vi "pwm_analog_digital.vi"() -> ()   [LabVIEW 2018]
uses:
  <vilib>/Instr/_visa.llb/VISA Configure Serial Port (Instr).vi
panel:
  in  "Boolean":bool
  out "concatenated string":string
  in  "Slide":dbl(slide) scale=0.0..255.0
  out "x = y?":bool
  in  "stop":bool
  out "Gauge":dbl(knob)
  in  "VISA resource name":refnum<visa-resource-name>
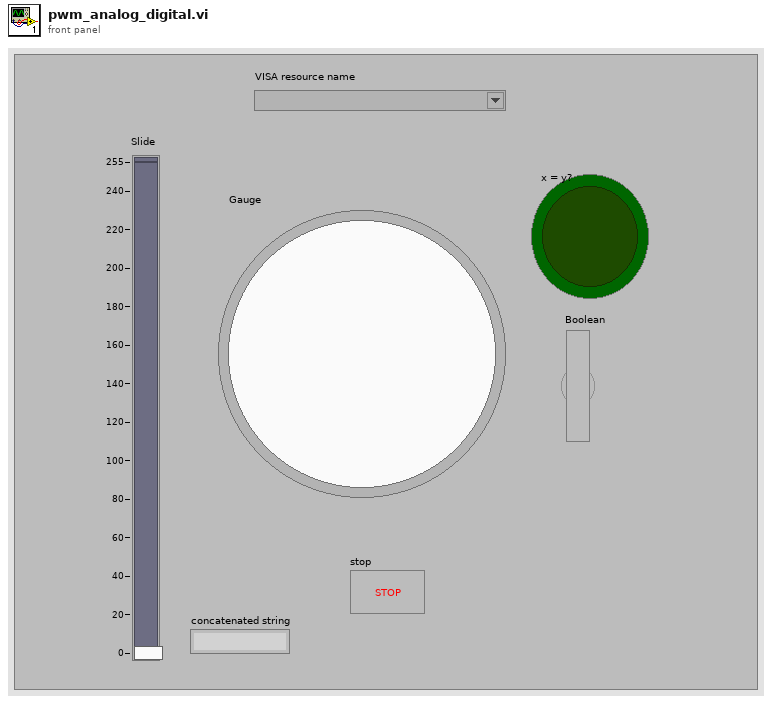
[diagram p1: front panel]
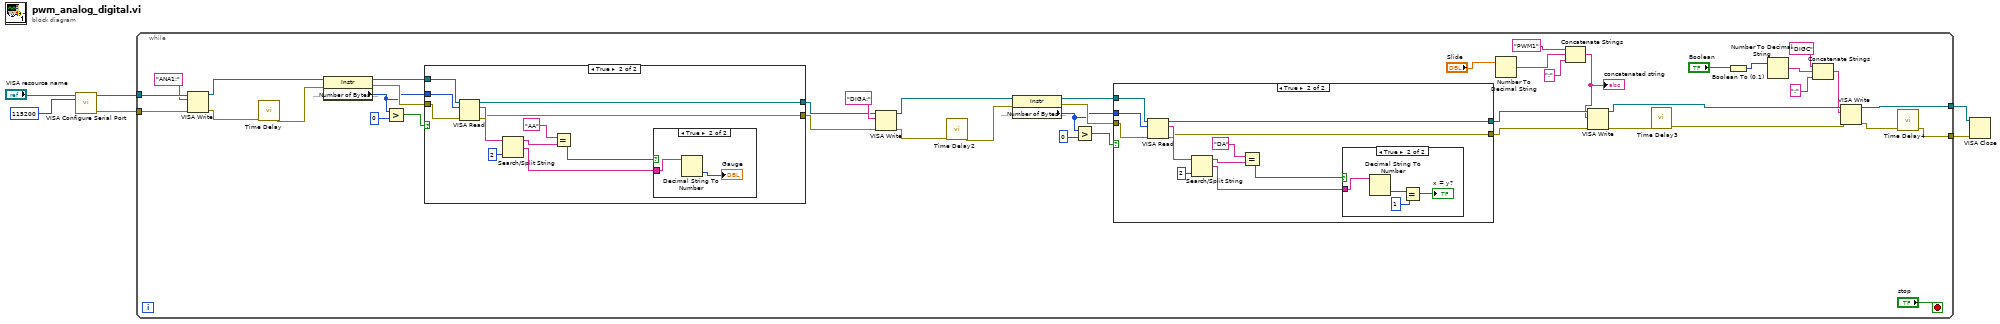
[diagram p0: block diagram]
diagram:
  n1 = call-poly "VISA Configure Serial Port"("VISA resource name"="VISA resource name", "baud rate (9600)"=u32 115200) -> ("VISA resource name out"=w4:refnum<visa-resource-name>, "error out"=w3:errorcluster)  [unwired: 12 in]
  n2 = while {
    tunnel: w4 -> [w48]
    tunnel: w3 -> [w47]
    tunnel: [w8] -> w2
    tunnel: [w7] -> w1
    stop <- "stop" stop-if-true
    n3 = VISA Write(VISA resource name=w48, write buffer="ANA1:", error in (no error)=w47) -> (VISA resource name out=w43:refnum<visa-resource-name>, error out=w45:errorcluster)  [unwired: 1 out]
    n4 = call "Time Delay"("error in (no error)"=w45) -> ("error out"=w44:errorcluster)  [unwired: 10 in]
    n5 = property class="Instr"(reference=w43, error in=w44) -> (reference out=w40:refnum<visa-resource-name>, error out=w39:errorcluster, "Serial Settings:Number of Bytes at Serial Port"=w38:u32)
    n6 = Greater?(x=w38, y=u32 0) -> (0:w41:bool)
    n7 = case shown="True" w41 {
      tunnel: w40 -> [w67 w78]
      tunnel: w39 -> [w66 w77]
      tunnel: w38 -> [_ w76]
      tunnel: [w67 w69] -> w27
      tunnel: [w66 w68] -> w26
      frame False {
      }
      frame True {
        n8 = VISA Read(VISA resource name=w78, byte count=w76, error in (no error)=w77) -> (VISA resource name out=w69:refnum<visa-resource-name>, read buffer=w74:string, error out=w68:errorcluster)  [unwired: 1 out]
        n9 = Search/Split String(string=w74, offset (0)=2) -> (substring before match=w73:string, match + rest of string=w70:string)  [unwired: 1 in, 1 out]
        n10 = Equal?(x="AA", y=w73) -> (x = y?=w71:bool)
        n11 = case shown="True" w71 {
          tunnel: w70 -> [_ w80]
          frame False {
          }
          frame True {
            n12 = Decimal String To Number(string=w80) -> (number=→"Gauge":i32)  [unwired: 2 in, 1 out]
          }
        }
      }
    }
    n13 = VISA Write(VISA resource name=w27, write buffer="DIGA:", error in (no error)=w26) -> (VISA resource name out=w34:refnum<visa-resource-name>, error out=w36:errorcluster)  [unwired: 1 out]
    n14 = call "Time Delay2"("error in (no error)"=w36) -> ("error out"=w35:errorcluster)  [unwired: 10 in]
    n15 = property class="Instr"(reference=w34, error in=w35) -> (reference out=w31:refnum<visa-resource-name>, error out=w30:errorcluster, "Serial Settings:Number of Bytes at Serial Port"=w29:u32)
    n16 = Greater?(x=w29, y=u32 0) -> (0:w32:bool)
    n17 = case shown="True" w32 {
      tunnel: w31 -> [w50 w61]
      tunnel: w30 -> [w49 w60]
      tunnel: w29 -> [_ w59]
      tunnel: [w50 w52] -> w24
      tunnel: [w49 w51] -> w25
      frame False {
      }
      frame True {
        n18 = VISA Read(VISA resource name=w61, byte count=w59, error in (no error)=w60) -> (VISA resource name out=w52:refnum<visa-resource-name>, read buffer=w57:string, error out=w51:errorcluster)  [unwired: 1 out]
        n19 = Search/Split String(string=w57, offset (0)=2) -> (substring before match=w56:string, match + rest of string=w53:string)  [unwired: 1 in, 1 out]
        n20 = Equal?(x="DA", y=w56) -> (x = y?=w54:bool)
        n21 = case shown="True" w54 {
          tunnel: w53 -> [_ w65]
          frame False {
          }
          frame True {
            n22 = Decimal String To Number(string=w65) -> (number=w64:i32)  [unwired: 2 in, 1 out]
            n23 = Equal?(x=w64, y=1) -> (x = y?=→"x = y?":bool)
          }
        }
      }
    }
    n24 = Number To Decimal String(number="Slide") -> (decimal integer string=w21:string)  [unwired: 1 in]
    n25 = Concatenate Strings("PWM1" ("string"), w21, ":" ("string")) -> (w19:string)
    "concatenated string" <- w19
    n26 = VISA Write(VISA resource name=w24, write buffer=w19, error in (no error)=w25) -> (VISA resource name out=w18:refnum<visa-resource-name>, error out=w17:errorcluster)  [unwired: 1 out]
    n27 = call "Time Delay3"("error in (no error)"=w17) -> ("error out"=w16:errorcluster)  [unwired: 10 in]
    n28 = Boolean To (0,1)(Boolean="Boolean") -> (0, 1=w14:i16)
    n29 = Number To Decimal String(number=w14) -> (decimal integer string=w12:string)  [unwired: 1 in]
    n30 = Concatenate Strings("DIGC" ("string"), w12, ":" ("string")) -> (w10:string)
    n31 = VISA Write(VISA resource name=w18, write buffer=w10, error in (no error)=w16) -> (VISA resource name out=w7:refnum<visa-resource-name>, error out=w9:errorcluster)  [unwired: 1 out]
    n32 = call "Time Delay4"("error in (no error)"=w9) -> ("error out"=w8:errorcluster)  [unwired: 10 in]
  }
  n33 = VISA Close(VISA resource name=w1, error in (no error)=w2) -> ()  [unwired: 1 out]
